vi "onFormatMQTTPacket.vi"(7 "PacketFormatter":refnum<class "PacketFormatter.lvclass">, 10 "packet":T1) -> (2 "String":string)   [LabVIEW 2013, in "MQTT Base.lvlib" / "PacketFormatter.lvclass"]
uses:
  PacketFormatter.lvclass
  DebuggingTerminal/Packet Arrival -- cluster.ctl
  <vilib>/LabVIEW Open Source Project/MQTT Control Packets/Control Packets/ControlPacket/ControlPacket.lvclass
  <vilib>/LabVIEW Open Source Project/MQTT Control Packets/Control Packets/ControlPacket/ControlPacket.lvclass/ControlPacket.ctl
  DebuggingTerminal/DebuggingTerminal.lvclass
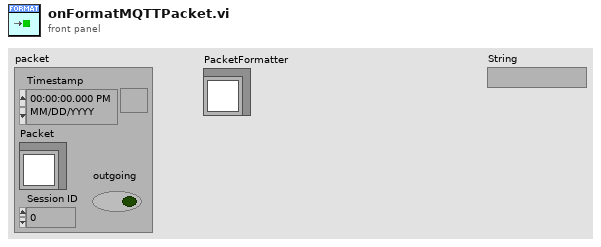
[diagram p1: front panel]
types:
  T1 = typedef "MQTT Base.lvlib/DebuggingTerminal.lvclass/Packet Arrival -- cluster.ctl" = cluster{"Timestamp":timestamp, "Packet":refnum<class "ControlPacket.lvclass">, "Session ID":i32, "outgoing":bool}
  T2 = typedef "MQTT_Control_Packets.lvlib/ControlPacket.lvclass/Control Packet Type -- enum.ctl" = enum16{"Reserved", "CONNECT", "CONNACK", "PUBLISH", "PUBACK", "PUBREC", "PUBREL", "PUBCOMP", "SUBSCRIBE", "SUBACK", "UNSUBSCRIBE", "UNSUBACK", "PINGREQ", "PINGRESP", "DISCONNECT", "AUTH"}
  T3 = typedef "MQTT_Control_Packets.lvlib/ControlPacket.lvclass/QualityOfService -- enum.ctl" = enum16{"0 (At Most Once)", "1 (At Least Once)", "2 (Exactly Once)"}
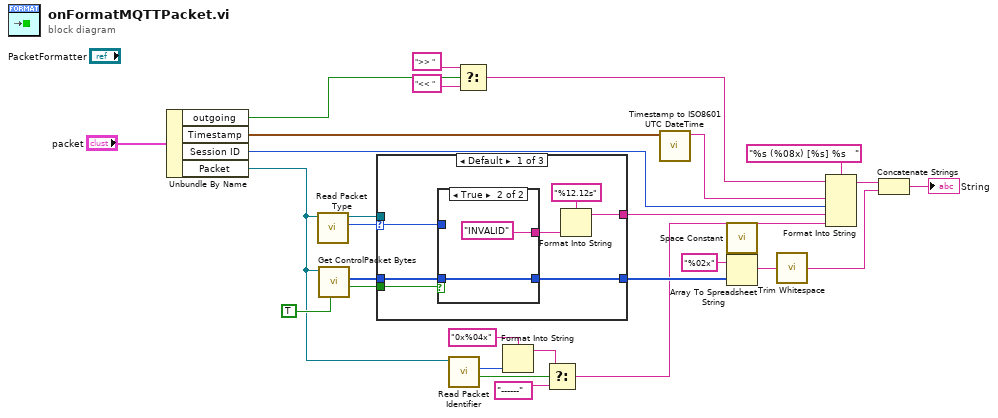
[diagram p0: block diagram]
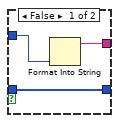
[diagram p2: hidden frame]
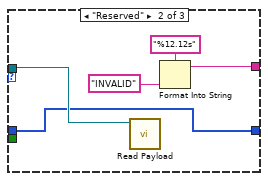
[diagram p3: hidden frame]
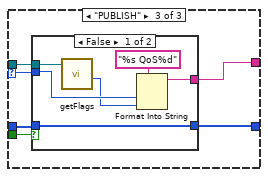
[diagram p4: hidden frame]
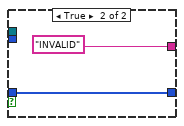
[diagram p5: hidden frame]
diagram:
  n1 = Unbundle By Name("packet") -> ("outgoing"=w2:bool, "Timestamp"=w22:timestamp, "Session ID"=w6:i32, "Packet"=w24:refnum<class "ControlPacket.lvclass">)
  n2 = call <vilib>:"Read Packet Type.vi"("ControlPacket in"=w24) -> ("Control Packet Type"=w26:T2, "ControlPacket out"=w10:refnum<class "ControlPacket.lvclass">)  [unwired: 9 in]
  n3 = call <vilib>:"Get ControlPacket Bytes.vi"("Validate? (F)"=TRUE, "ControlPacket"=w24) -> ("Packet invalid"=w27:bool, "Bytes Stream"=w25:u8[])  [unwired: 6 in, 2 out]
  n4 = case shown="Default" w26 {
    selector: w26 -> [w30 _ w52]
    tunnel: [w35 w45 w48] -> w11
    tunnel: w10 -> [_ w43 w47]
    tunnel: [w33 w42 w49] -> w23
    tunnel: w25 -> [w32 w42 w51]
    tunnel: w27 -> [w34 _ w50]
    frame Default {
      n5 = case shown="True" w34 {
        tunnel: [w39 w41] -> w33
        tunnel: w32 -> [w39 w41]
        tunnel: [w37 "INVALID" ("format string")] -> w31
        tunnel: w30 -> [w38 _]
        frame False {
          n6 = Format Into String(w38) -> (resulting string=w37:string)  [unwired: 3 in, 1 out]
        }
        frame True {
        }
      }
      n7 = Format Into String(format string="%12.12s", w31) -> (resulting string=w35:string)  [unwired: 2 in, 1 out]
    }
    frame "Reserved" {
      n8 = call <vilib>:"Read Payload.vi"("ControlPacket in"=w43) -> ()  [unwired: 9 in, 2 out]
      n9 = Format Into String(format string="%12.12s", "INVALID" ("format string")) -> (resulting string=w45:string)  [unwired: 2 in, 1 out]
    }
    frame "PUBLISH" {
      n10 = case shown="False" w50 {
        tunnel: [w58 w60] -> w49
        tunnel: w51 -> [w58 w60]
        tunnel: [w56 "INVALID" ("format string")] -> w48
        tunnel: w52 -> [w57 _]
        tunnel: w47 -> [w54 _]
        frame False {
          n11 = call-dynamic "getFlags.vi"("ControlPacket in"=w54) -> ("QoS"=w53:T3)  [unwired: 7 in, 3 out]
          n12 = Format Into String(format string="%s QoS%d", w57, w53) -> (resulting string=w56:string)  [unwired: 2 in, 1 out]
        }
        frame True {
        }
      }
    }
  }
  n13 = call <vilib>:"Read Packet Identifier.vi"("ControlPacket in"=w24) -> ("Has Packet Identifier"=w20:bool, "Packet Identifier"=w18:u16)  [unwired: 8 in, 1 out]
  n14 = Select(t=">> " ("format string"), s=w2, f="<< " ("format string")) -> (s? t:f=w1:string)
  n15 = Format Into String(format string="0x%04x", w18) -> (resulting string=w16:string)  [unwired: 2 in, 1 out]
  n16 = Select(t=w16, s=w20, f="------" ("format string")) -> (s? t:f=w21:string)
  n17 = call <vilib>:"Timestamp to ISO8601 UTC DateTime.vi"("Timestamp (now)"=w22) -> ("ISO8601 UTC DateTime"=w7:string)  [unwired: 10 in]
  n18 = call <vilib>:"Space Constant.vi"() -> ("String"=w13:string)
  n19 = Array To Spreadsheet String(delimiter (Tab)=w13, array=w23, 3:"%02x" ("format string")) -> (spreadsheet string=w12:string)
  n20 = call <vilib>:"Trim Whitespace.vi"("string"=w12) -> ("trimmed string"=w15:string)  [unwired: 1 in]
  n21 = Format Into String(format string="%s (%08x) [%s] %s   ", initial string=w1, w7, w6, w11, w21) -> (resulting string=w9:string)  [unwired: 1 in, 1 out]
  n22 = Concatenate Strings(w9, w15) -> (→"String":string)
